vi "display_plot.vi"(0 "Input Data":cluster{"all rows":dbl[], "all rows":dbl[]}(graph), 1 "X Scale.Name Label.Text":string, 2 "Y Scale.Name Label.Text":string, 3 "FileName":string, 6 "xValues":i32, 8 "yValues":i32, 10 "File Path":path) -> ()   [LabVIEW 2019]
uses:
  <vilib>/Analysis/Matrix/Numeric/Conversions/Array To Matrix - RA2.vi
  <vilib>/Analysis/Matrix/Numeric/Conversions/Matrix To Array - RM.vi
  <vilib>/Analysis/Matrix/NI_Matrix.lvlib
panel:
  out "Output Graph":cluster{"all rows":dbl[], "all rows":dbl[]}(graph)
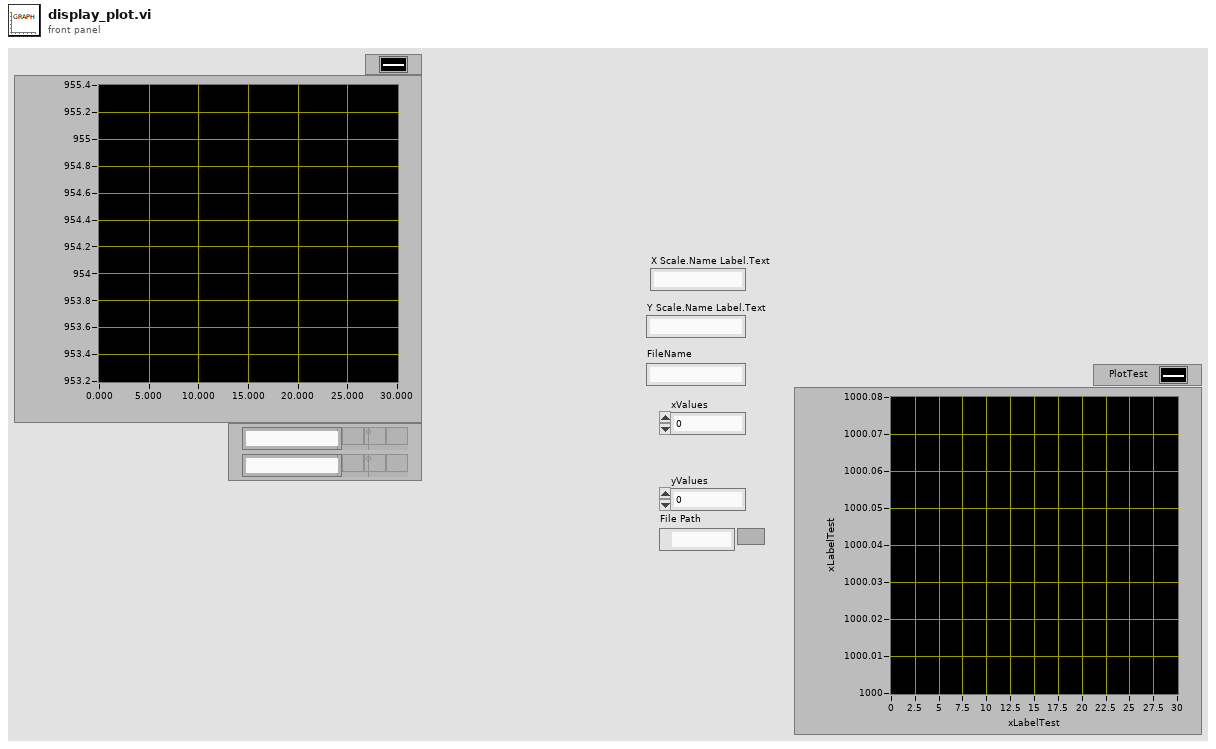
[diagram p1: front panel]
types:
  T1 = typedef "NI_Matrix.lvlib/RealMatrix.ctl" = dbl[][]
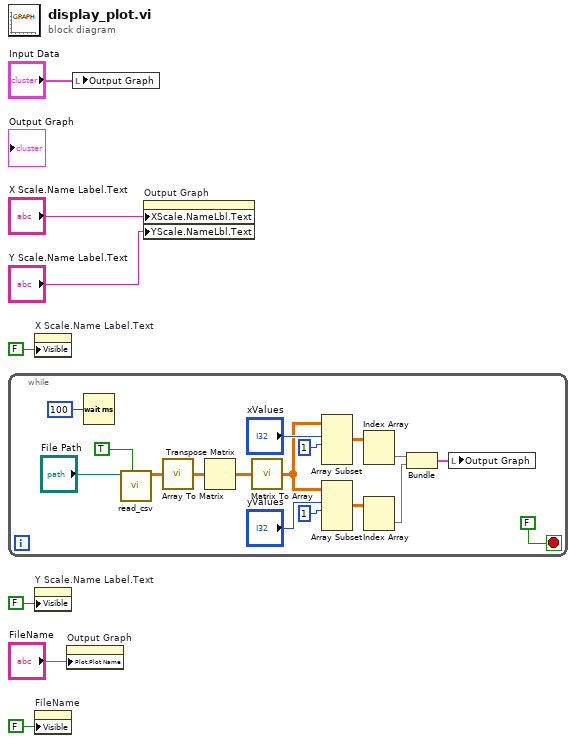
[diagram p0: block diagram]
diagram:
  n1 = while {
    stop <- FALSE stop-if-true
    n2 = Wait (ms)(milliseconds to wait=u32 100) -> ()  [unwired: 1 out]
    n3 = call "read_csv.vi"("Read"=TRUE, "Read File:"="File Path") -> ("File Data"=w14:T1)  [unwired: 9 in]
    n4 = call-poly <vilib>:"Array To Matrix.vi"("Real 2D Array"=w14) -> ("Real Matrix"=w23:T1)
    n5 = Transpose Matrix(1:w23) -> (0:w24:T1)
    n6 = call-poly <vilib>:"Matrix To Array.vi"("Real Matrix"=w24) -> ("Real 2D Array"=w20:dbl[][])
    n7 = Array Subset(array=w20, index (row)="xValues", length (row)=1 ("length")) -> (w19:dbl[][])  [unwired: 2 in]
    n8 = Array Subset(array=w20, index (row)="yValues", length (row)=1 ("length")) -> (w17:dbl[][])  [unwired: 2 in]
    n9 = Index Array(array=w19) -> (element=w18:dbl[])  [unwired: 2 in]
    n10 = Index Array(array=w17) -> (element=w16:dbl[])  [unwired: 2 in]
    n11 = Bundle(w18, w16) -> (w9:cluster{dbl[], dbl[]})  [unwired: 1 in]
    n12 = local write "Output Graph"(w9) -> ()
  }
  n13 = property on="X Scale.Name Label.Text" class="Str"("Visible"=FALSE) -> ()  [unwired: 2 in, 2 out]
  n14 = property on="Y Scale.Name Label.Text" class="Str"("Visible"=FALSE) -> ()  [unwired: 2 in, 2 out]
  n15 = property on="FileName" class="Str"("Visible"=FALSE) -> ()  [unwired: 2 in, 2 out]
  n16 = property on="Output Graph" class="XYGraph (strict)"("Plot.Plot Name"="FileName") -> ()  [unwired: 2 in, 2 out]
  n17 = local write "Output Graph"("Input Data") -> ()
  n18 = property on="Output Graph" class="XYGraph (strict)"("XScale.NameLbl.Text"="X Scale.Name Label.Text", "YScale.NameLbl.Text"="Y Scale.Name Label.Text") -> ()  [unwired: 2 in, 2 out]
